vi "Main.vi"() -> ()   [LabVIEW 2023]
doc: "This template is for the Queued Message Handler design pattern.\n\nThe Event Handling Loop generates messages based on user interface actions.\n\nThe Message Handling Loop processes messages generated by the Event Handling Loop, or by other messages. The messages are string values, so new messages can be added easily to the Message Cases case structure in the Message Handling Loop. Each message cluster can also provide an optional value for Message Data, which is a variant that can be converted to whatever message-specific data is required."
uses:
  controls/JogParameters.ctl
  controls/MoveParameters.ctl
  controls/UI Data.ctl
  support/Message Queue/Enqueue Message (Single).vi
  chem-maldonado-motion-controller-api/GlobalVarsNetwork.vi
  <vilib>/Utility/error.llb/Error Cluster From Error Code.vi
  <vilib>/ErrorRing/Error Ring.xnode
  support/Message Queue/Message Queue.lvlib
  support/User Event - Stop/User Event - Stop.lvlib
panel:
  in  "Perform Home Routine":T1
  in  "Change Encoder Direction":T2
  out "Encoder Directions":T3
  out "X position (µm)":dbl
  out "X position (mm)":dbl
  out "Y position (µm)":dbl
  out "Y position (mm)":dbl
  out "Z position (µm)":dbl
  out "Z position (mm)":dbl
  in  "Jog Z":T4 {"Speed" min=0.0 max=1500.0}
  in  "Jog Y":T4 {"Speed" min=0.0 max=1500.0}
  in  "Move Z":T5 {"Speed" min=0.0 max=1500.0}
  in  "Move Y":T5 {"Speed" min=0.0 max=1500.0}
  in  "Move X":T5 {"Speed" min=0.0 max=1500.0}
  in  "Jog X":T4 {"Speed" min=0.0 max=1500.0}
  in  "Stop Motion":bool
  out "Action":string
  in  "Exit VI":bool
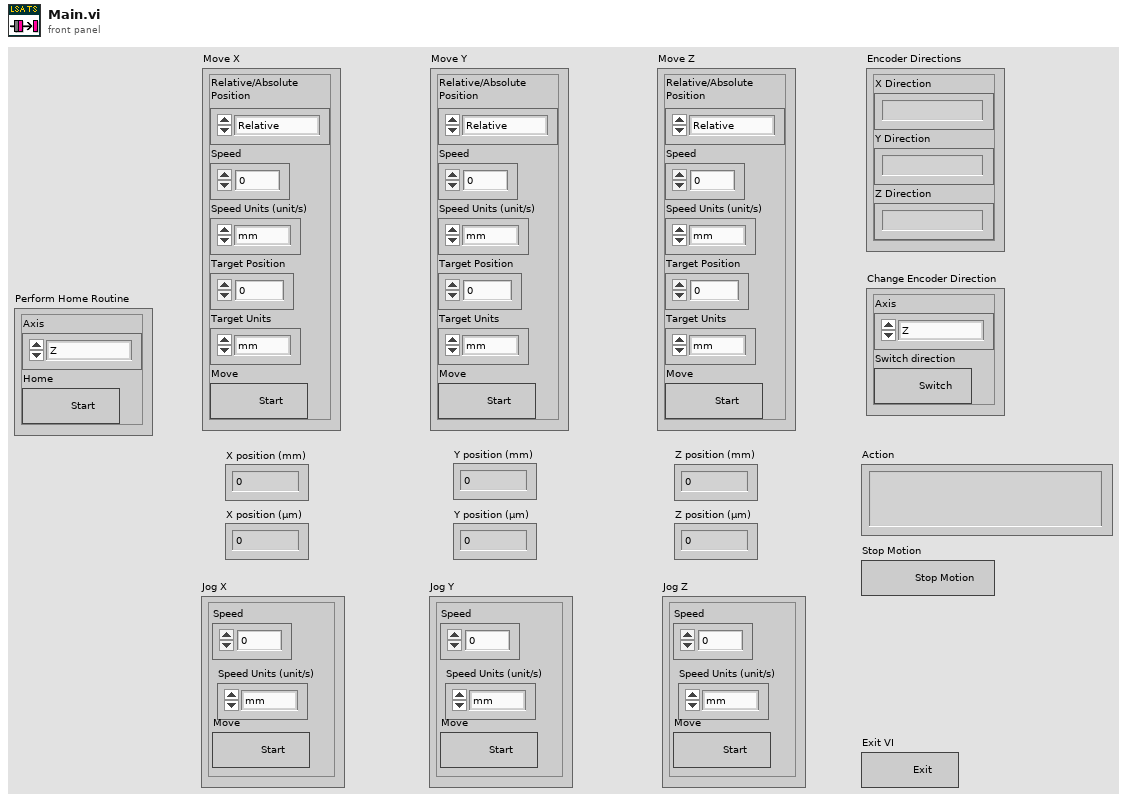
[diagram p1: front panel]
types:
  T1 = cluster{"Axis":enum16{"Z", "Y", "X"}, "Home":bool}
  T2 = cluster{"Axis":enum16{"Z", "Y", "X"}, "Switch direction":bool}
  T3 = cluster{"X Direction":string, "Y Direction":string, "Z Direction":string}
  T4 = typedef "JogParameters.ctl" = cluster{"Speed":dbl, "Speed Units (unit/s)":enum16{"mm", "µm"}, "Move":bool}
  T5 = typedef "MoveParameters.ctl" = cluster{"Relative/Absolute\nPosition":enum16{"Relative", "Absolute"}, "Speed":dbl, "Speed Units (unit/s)":enum16{"mm", "µm"}, "Target Position":dbl, "Target Units":enum16{"mm", "µm"}, "Move":bool}
  T6 = typedef "UI Data.ctl" = cluster{"Boolean <Replace Me>":bool, "String <Replace Me>":string, "Numeric <Replace Me>":dbl, "Do Something Ref":refnum<vi>, "Do Something Else Ref":refnum<vi>, "Data Display Ref":refnum<vi>, "Exit Button Ref":refnum<vi>, "StopMotion Button Ref":refnum<vi>}
  T7 = typedef "Message Queue.lvlib/All Message Queues.ctl" = cluster{"UI":refnum<queue>}
  T8 = cluster{"XY_IP_ADDRESS":string, "Z_IP_ADDRESS":string, "Port":u16, "connection refnum x,y":refnum<k5>, "connection refnum z":refnum<k5>}
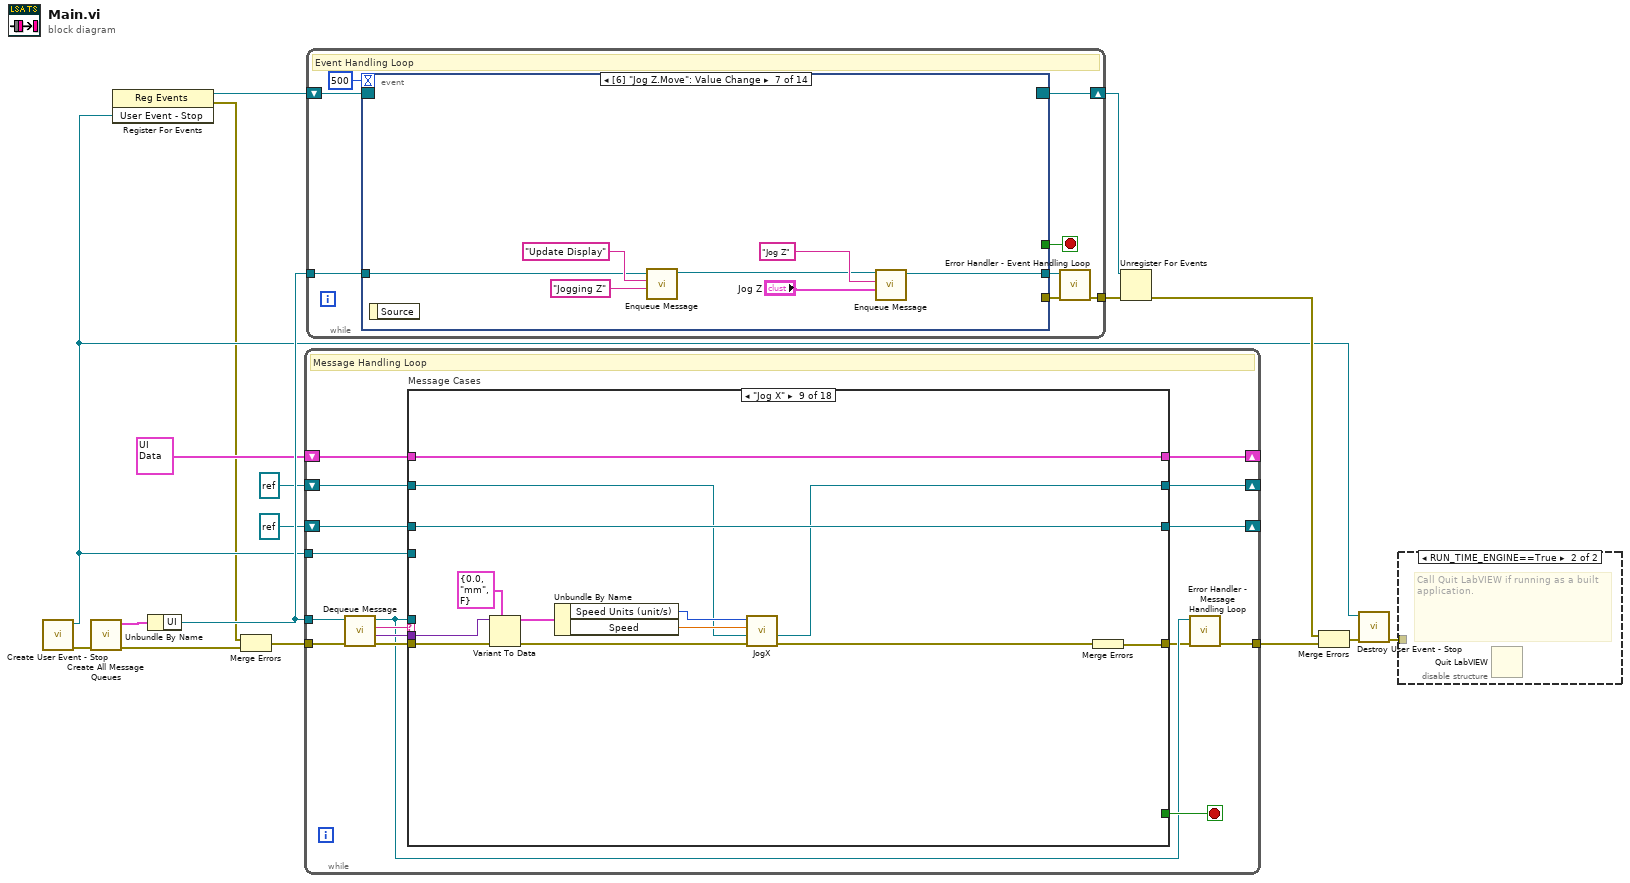
[diagram p0: block diagram]
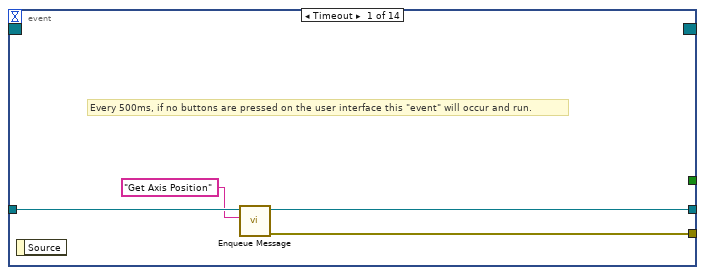
[diagram p3: hidden frame]
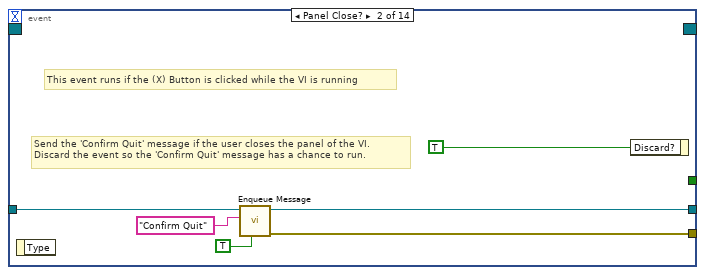
[diagram p4: hidden frame]
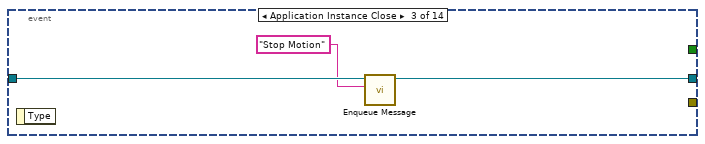
[diagram p5: hidden frame]
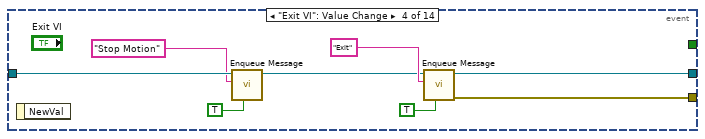
[diagram p6: hidden frame]
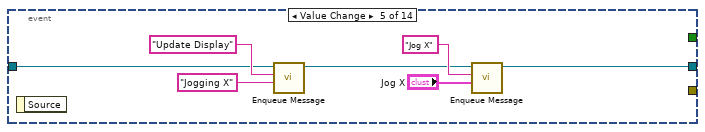
[diagram p7: hidden frame]
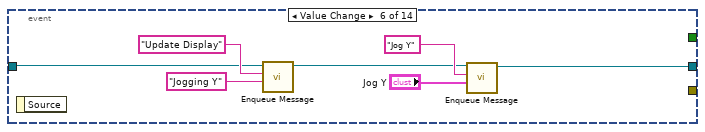
[diagram p8: hidden frame]
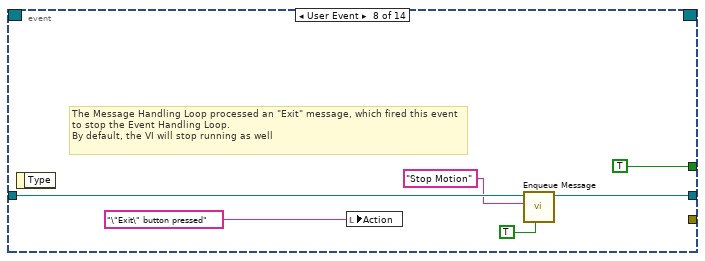
[diagram p9: hidden frame]
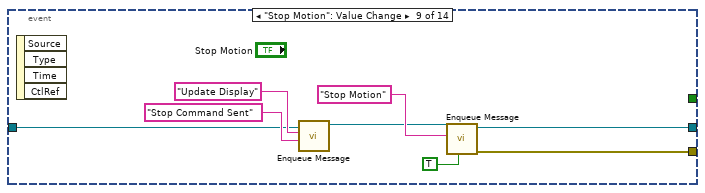
[diagram p10: hidden frame]
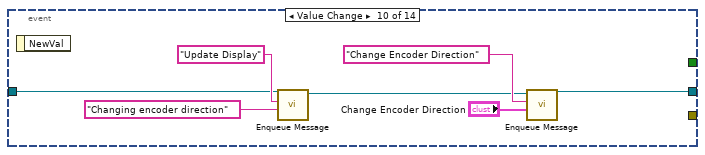
[diagram p11: hidden frame]
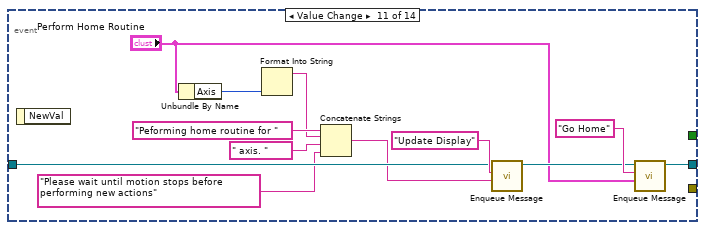
[diagram p12: hidden frame]
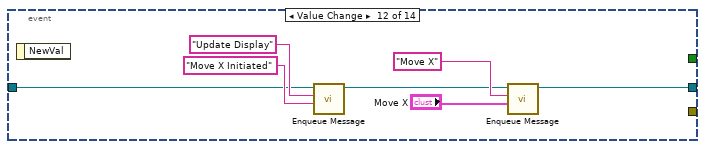
[diagram p13: hidden frame]
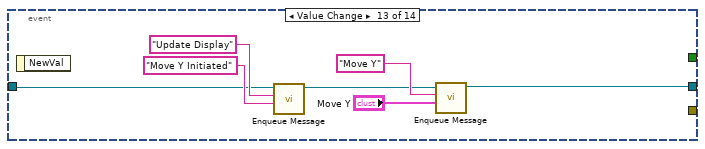
[diagram p14: hidden frame]
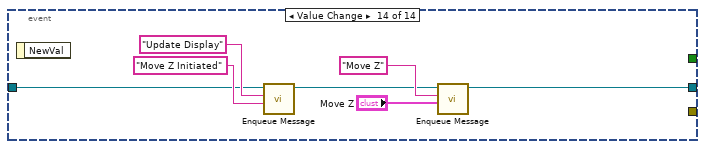
[diagram p15: hidden frame]
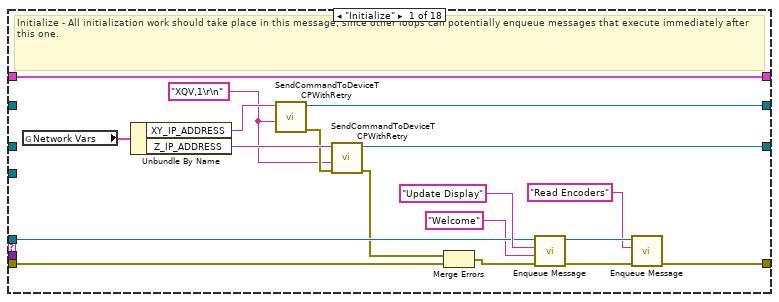
[diagram p16: hidden frame]
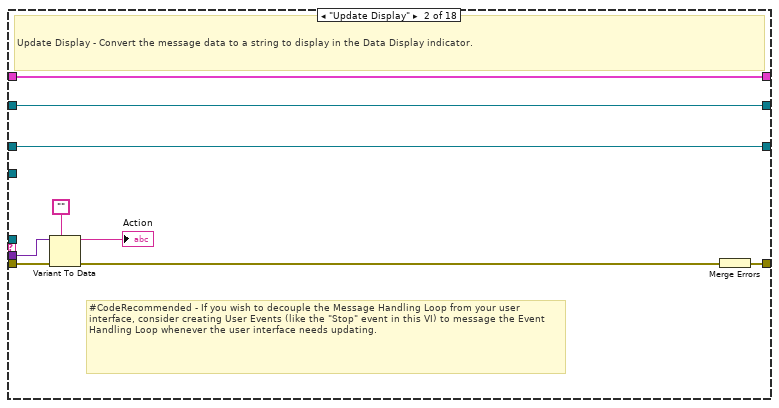
[diagram p17: hidden frame]
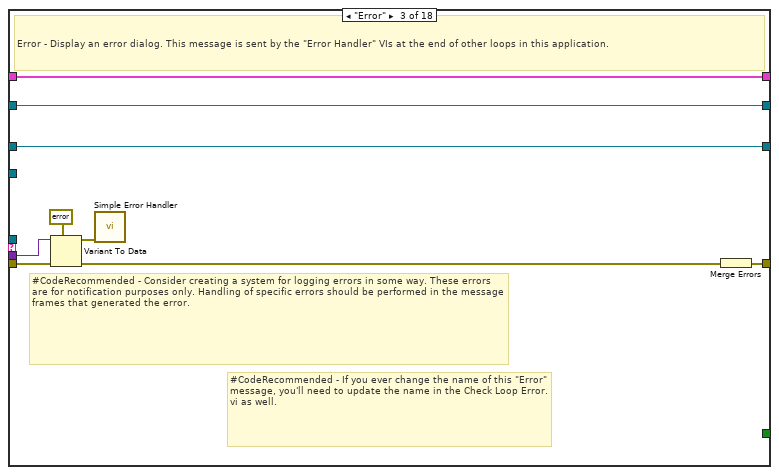
[diagram p18: hidden frame]
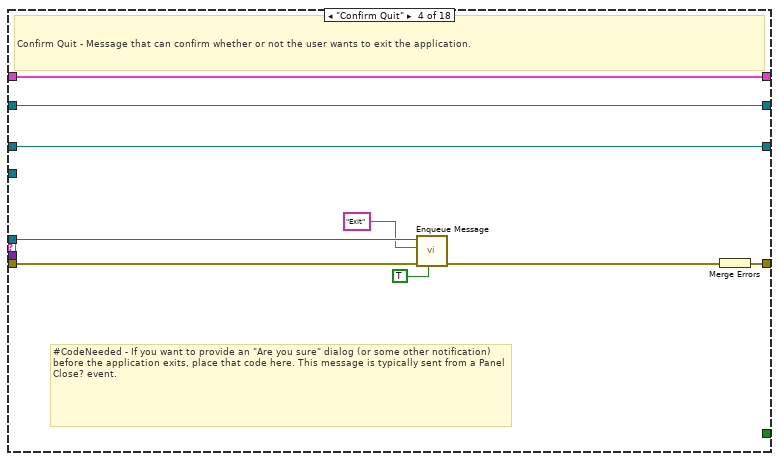
[diagram p19: hidden frame]
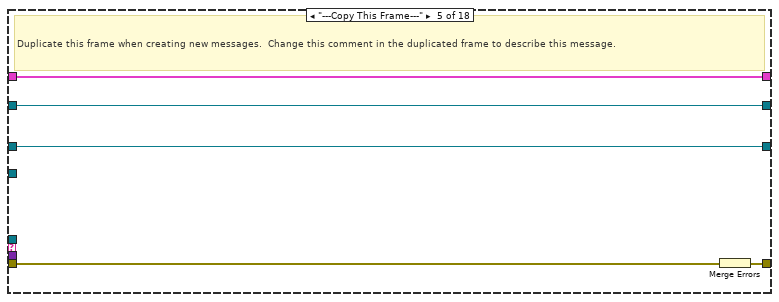
[diagram p20: hidden frame]
diagram:
  n1 = call "Create User Event - Stop.vi"() -> ("error out"=w13:errorcluster, "User Event - Stop"=w5:refnum<user-event>)  [unwired: 10 in]
  n2 = call "Create All Message Queues.vi"("error in (no error)"=w13) -> ("error out"=w17:errorcluster, "Message Queues out"=w16:T7)  [unwired: 9 in]
  n3 = register-events(w5) -> (reference out=w6:refnum<event-registration>, error out=w3:errorcluster)  [unwired: 2 in]
  n4 = Unbundle By Name(w16) -> ("UI"=w14:refnum<queue>)
  n5 = Merge Errors(w3, w17) -> (w4:errorcluster)
  n6 = while {
    tunnel: w14 -> [w25]
    shift-right: [w32] -> _
    shift-left: T6 {"Boolean <Replace Me>"=FALSE, "String <Replace Me>"="", "Numeric <Replace Me>"=0.0, "Do Something Ref"=refnum, "Do Something Else Ref"=refnum, "Data Display Ref"=refnum, "Exit Button Ref"=refnum, "StopMotion Button Ref"=refnum} ("Data Cluster") -> [w33]
    tunnel: w5 -> [w30]
    tunnel: w4 -> [w29]
    tunnel: [w23] -> w15
    shift-right: [w21] -> _
    shift-left: refnum<k5> refnum ("connection refnum out") -> [w20]
    shift-right: [w19] -> _
    shift-left: refnum<k5> refnum ("connection refnum out") -> [w18]
    stop <- w31 stop-if-true
    # "Message Handling Loop"
    n7 = call "Dequeue Message.vi"("error in (no error)"=w29, "Message Queue"=w25) -> ("error out"=w28:errorcluster, "Message Data"=w26:variant, "Message"=w27:string, "dup Message Queue"=w24:refnum<queue>)  [unwired: 6 in]
    n8 = case "Message Cases" shown="\"Jog X\"" w27 {
      selector: w27 -> [_ _ _ _ _ _ _ _ _ _ _ _ _ _ _ _ w302 _]
      tunnel: w24 -> [w50 _ _ w74 _ _ _ _ _ _ _ _ w199 w229 _ w299 _ _]
      tunnel: w28 -> [w42 w58 w69 w78 w83 w91 w105 w127 w142 w152 w165 w190 w205 w233 w265 w292 _ w318]
      tunnel: [w36 w59 w63 w76 w81 w88 w104 w129 w135 w148 w161 w189 w200 w235 w249 w295 w303 w317] -> w22
      tunnel: w33 -> [w48 w60 w68 w77 w82 w99 w114 w130 w143 w156 w169 w191 w217 w236 w266 w298 w304 w319]
      tunnel: [w48 w60 w68 w77 w82 w99 w114 w130 w143 w156 w169 w191 w217 w236 w266 w298 w304 w319] -> w32
      tunnel: [_ _ _ _ _ _ _ _ _ _ _ _ _ _ _ TRUE _ _] -> w31
      tunnel: w26 -> [_ w57 w67 _ _ w98 w112 w126 w139 w155 w166 _ _ w232 w263 w289 _ _]
      tunnel: w30 -> [_ _ _ _ _ _ _ _ _ _ _ _ _ _ _ w294 _ _]
      tunnel: [w40 w53 w62 w71 w80 w84 w100 w116 w131 w144 w157 w170 w207 w219 w253 w285 w300 w313] -> w21
      tunnel: w20 -> [_ w53 w62 w71 w80 w85 w101 w116 w132 w145 w157 w171 w209 w227 w256 w288 w300 w314]
      tunnel: [w39 w52 w61 w70 w79 w86 w102 w115 w133 w146 w158 w173 w206 w218 w251 w286 w301 w312] -> w19
      tunnel: w18 -> [_ w52 w61 w70 w79 w86 w102 w117 w133 w146 w159 w174 w210 w226 w252 w287 w301 w315]
      frame "Initialize" {
        w43 = "XQV,1\r\n" ("str command")
        # "Initialize - All initialization work should take place in this message, since other loops can potentially enqueue messages that execute immediately after this one."
        n9 = global read "GlobalVarsNetwork.vi" "Network Vars"() -> (w47:T8)
        n10 = Unbundle By Name(w47) -> ("XY_IP_ADDRESS"=w46:string, "Z_IP_ADDRESS"=w45:string)
        n11 = call "SendCommandToDeviceTCPWithRetry.vi"("str command"=w43, "IP address"=w46) -> ("error out"=w44:errorcluster, "connection refnum out"=w40:refnum<k5>)  [unwired: 6 in, 2 out]
        n12 = call "SendCommandToDeviceTCPWithRetry.vi"("error in"=w44, "str command"=w43, "IP address"=w45) -> ("error out"=w38:errorcluster, "connection refnum out"=w39:refnum<k5>)  [unwired: 5 in, 2 out]
        n13 = Merge Errors(w38, w42) -> (w41:errorcluster)
        n14 = call-poly "Enqueue Message.vi"("error in (no error)"=w41, "Message Data"="Welcome" ("Initial Message"), "Message"="Update Display", "Message Queue"=w50) -> ("error out"=w37:errorcluster, "dup Message Queue"=w35:refnum<queue>)  [unwired: 6 in]
        n15 = call-poly "Enqueue Message.vi"("error in (no error)"=w37, "Message"="Read Encoders", "Message Queue"=w35) -> ("error out"=w36:errorcluster)  [unwired: 7 in, 1 out]
      }
      frame "Update Display" {
        # "#CodeRecommended - If you wish to decouple the Message Handling Loop from your user interface, consider creating User Events (like the \"Stop\" event in this VI) to message the Event Handling Loop whenever the user interface needs updating."
        # "Update Display - Convert the message data to a string to display in the Data Display indicator."
        n16 = Variant To Data(error in=w58, type="", Variant=w57) -> (data=→"Action":string, error out=w55:errorcluster)
        n17 = Merge Errors(w55) -> (w59:errorcluster)
      }
      frame "Error" {
        # "#CodeRecommended - If you ever change the name of this \"Error\" message, you'll need to update the name in the Check Loop Error.vi as well."
        # "#CodeRecommended - Consider creating a system for logging errors in some way. These errors are for notification purposes only. Handling of specific errors should be performed in the message frames that generated the error."
        # "Error - Display an error dialog. This message is sent by the \"Error Handler\" VIs at the end of other loops in this application."
        n18 = Variant To Data(error in=w69, type=errorcluster {"status"=FALSE, "code"=0, "source"=""} ("error constant"), Variant=w67) -> (data=w65:errorcluster, error out=w64:errorcluster)
        n19 = call <vilib>:"Simple Error Handler.vi"("error in (no error)"=w65) -> ()  [unwired: 4 in, 5 out]
        n20 = Merge Errors(w64) -> (w63:errorcluster)
      }
      frame "Confirm Quit" {
        # "#CodeNeeded - If you want to provide an \"Are you sure\" dialog (or some other notification) before the application exits, place that code here. This message is typically sent from a Panel Close? event."
        # "Confirm Quit - Message that can confirm whether or not the user wants to exit the application."
        n21 = call-poly "Enqueue Message.vi"("Priority Message? (F)"=TRUE, "error in (no error)"=w78, "Message"="Exit", "Message Queue"=w74) -> ("error out"=w75:errorcluster)  [unwired: 6 in, 1 out]
        n22 = Merge Errors(w75) -> (w76:errorcluster)
      }
      frame "---Copy This Frame---" {
        # "Duplicate this frame when creating new messages.  Change this comment in the duplicated frame to describe this message."
        n23 = Merge Errors(w83) -> (w81:errorcluster)
      }
      frame "Move X" {
        n24 = Variant To Data(error in=w91, type=T5 {"Relative/Absolute\nPosition"=enum."Relative", "Speed"=0.0, "Speed Units (unit/s)"=enum."mm", "Target Position"=0.0, "Target Units"=enum."mm", "Move"=FALSE} ("Move Parameters X"), Variant=w98) -> (data=w97:T5, error out=w90:errorcluster)
        n25 = Unbundle By Name(w97) -> ("Relative/Absolute\nPosition"=w96:enum16{"Relative", "Absolute"}, "Speed"=w95:dbl, "Speed Units (unit/s)"=w94:enum16{"mm", "µm"}, "Target Position"=w93:dbl, "Target Units"=w92:enum16{"mm", "µm"})
        n26 = call "MoveX.vi"("Speed (units/s)"=w95, "Relative/Absolute\nPosition"=w96, "connection refnum in"=w85, "Speed Units"=w94, "Target Position"=w93, "Target Units"=w92, "error in"=w90) -> ("connection refnum out xy"=w84:refnum<k5>, "error out"=w87:errorcluster)  [unwired: 6 in, 1 out]
        n27 = Merge Errors(w87) -> (w88:errorcluster)
      }
      frame "Move Y" {
        # "Duplicate this frame when creating new messages.  Change this comment in the duplicated frame to describe this message."
        n28 = Variant To Data(type=T5 {"Relative/Absolute\nPosition"=enum."Relative", "Speed"=0.0, "Speed Units (unit/s)"=enum."mm", "Target Position"=0.0, "Target Units"=enum."mm", "Move"=FALSE} ("Move Parameters Y"), Variant=w112) -> (data=w111:T5)  [unwired: 1 in, 1 out]
        n29 = Unbundle By Name(w111) -> ("Relative/Absolute\nPosition"=w110:enum16{"Relative", "Absolute"}, "Speed"=w109:dbl, "Speed Units (unit/s)"=w108:enum16{"mm", "µm"}, "Target Position"=w107:dbl, "Target Units"=w106:enum16{"mm", "µm"})
        n30 = call "MoveY.vi"("Speed (unit/s)"=w109, "Relative/Absolute\nPosition"=w110, "connection refnum in"=w101, "Speed Units"=w108, "Target Position"=w107, "Target Units"=w106, "error in"=w105) -> ("connection refnum out xy"=w100:refnum<k5>, "error out"=w103:errorcluster)  [unwired: 6 in, 1 out]
        n31 = Merge Errors(w103) -> (w104:errorcluster)
      }
      frame "Move Z" {
        # "Duplicate this frame when creating new messages.  Change this comment in the duplicated frame to describe this message."
        n32 = Variant To Data(error in=w127, type=T5 {"Relative/Absolute\nPosition"=enum."Relative", "Speed"=0.0, "Speed Units (unit/s)"=enum."mm", "Target Position"=0.0, "Target Units"=enum."mm", "Move"=FALSE} ("Move Parameters Z"), Variant=w126) -> (data=w125:T5, error out=w119:errorcluster)
        n33 = Unbundle By Name(w125) -> ("Relative/Absolute\nPosition"=w124:enum16{"Relative", "Absolute"}, "Speed"=w123:dbl, "Speed Units (unit/s)"=w122:enum16{"mm", "µm"}, "Target Position"=w121:dbl, "Target Units"=w120:enum16{"mm", "µm"})
        n34 = call "MoveZ.vi"("Speed (unit/s)"=w123, "Relative/Absolute\nPosition"=w124, "connection refnum in"=w117, "Speed Units"=w122, "Target Position"=w121, "Target Units"=w120, "error in"=w119) -> ("connection refnum out z"=w115:refnum<k5>, "error out"=w118:errorcluster)  [unwired: 6 in, 1 out]
        n35 = Merge Errors(w118) -> (w129:errorcluster)
      }
      frame "Jog X" {
        n36 = Variant To Data(error in=w142, type=T4 {"Speed"=0.0, "Speed Units (unit/s)"=enum."mm", "Move"=FALSE} ("Jog X"), Variant=w139) -> (data=w138:T4, error out=w141:errorcluster)
        n37 = Unbundle By Name(w138) -> ("Speed Units (unit/s)"=w136:enum16{"mm", "µm"}, "Speed"=w137:dbl)
        n38 = call "JogX.vi"("error in"=w141, "connection refnum in"=w132, "Speed (units/s)"=w137, "Units"=w136) -> ("error out"=w134:errorcluster, "connection refnum out"=w131:refnum<k5>)  [unwired: 6 in]
        n39 = Merge Errors(w134) -> (w135:errorcluster)
      }
      frame "Jog Y" {
        n40 = Variant To Data(error in=w152, type=T4 {"Speed"=0.0, "Speed Units (unit/s)"=enum."mm", "Move"=FALSE} ("Jog X"), Variant=w155) -> (data=w153:T4, error out=w149:errorcluster)
        n41 = Unbundle By Name(w153) -> ("Speed Units (unit/s)"=w150:enum16{"mm", "µm"}, "Speed"=w151:dbl)
        n42 = call "JogY.vi"("error in"=w149, "connection refnum in"=w145, "Speed (units/s)"=w151, "Units"=w150) -> ("error out"=w147:errorcluster, "connection refnum out xy"=w144:refnum<k5>)  [unwired: 6 in]
        n43 = Merge Errors(w147) -> (w148:errorcluster)
      }
      frame "Jog Z" {
        n44 = Variant To Data(error in=w165, type=T4 {"Speed"=0.0, "Speed Units (unit/s)"=enum."mm", "Move"=FALSE} ("Jog X"), Variant=w166) -> (data=w168:T4, error out=w164:errorcluster)
        n45 = Unbundle By Name(w168) -> ("Speed Units (unit/s)"=w162:enum16{"mm", "µm"}, "Speed"=w163:dbl)
        n46 = call "JogZ.vi"("error in"=w164, "connection refnum in"=w159, "Speed (units/s)"=w163, "Units"=w162) -> ("error out"=w160:errorcluster, "connection refnum out z"=w158:refnum<k5>)  [unwired: 6 in]
        n47 = Merge Errors(w160) -> (w161:errorcluster)
      }
      frame "Get Axis Position" {
        n48 = call "GetAxisPosition.vi"("Axis"=enum16{"Z", "Y", "X"}."Z", "connection refnum in"=w174, "error in"=w190) -> ("connection refnum out"=w173:refnum<k5>, "numeric result"=w186:i32, "error out"=w188:errorcluster)  [unwired: 1 out]
        n49 = call "CountsToUnit.vi"("Counts"=w186) -> ("mm"=→"Z position (mm)":dbl, "µm"=→"Z position (µm)":dbl)  [unwired: 1 in, 1 out]
        n50 = call "GetAxisPosition.vi"("Axis"=enum16{"Z", "Y", "X"}."Y", "connection refnum in"=w171, "error in"=w188) -> ("connection refnum out"=w172:refnum<k5>, "numeric result"=w185:i32, "error out"=w187:errorcluster)  [unwired: 1 out]
        n51 = call "CountsToUnit.vi"("Counts"=w185) -> ("mm"=→"Y position (mm)":dbl, "µm"=→"Y position (µm)":dbl)  [unwired: 1 in, 1 out]
        n52 = call "GetAxisPosition.vi"("Axis"=enum16{"Z", "Y", "X"}."X", "connection refnum in"=w172, "error in"=w187) -> ("connection refnum out"=w170:refnum<k5>, "numeric result"=w184:i32, "error out"=w189:errorcluster)  [unwired: 1 out]
        n53 = call "CountsToUnit.vi"("Counts"=w184) -> ("mm"=→"X position (mm)":dbl, "µm"=→"X position (µm)":dbl)  [unwired: 1 in, 1 out]
      }
      frame "Read Encoders" {
        n54 = global read "GlobalVarsNetwork.vi" "Network Vars"() -> (w196:T8)
        n55 = Unbundle By Name(w196) -> ("XY_IP_ADDRESS"=w195:string, "Z_IP_ADDRESS"=w194:string)
        n56 = call "ReadEncoderDirection.vi"("error in"=w205, "IP address"=w195, "Axis"=enum16{"Z", "Y", "X"}."X", "connection refnum in"=w209) -> ("error out"=w216:errorcluster, "Encoder Direction"=w204:string, "connection refnum out"=w208:refnum<k5>)  [unwired: 4 in, 1 out]
        n57 = call "ReadEncoderDirection.vi"("error in"=w216, "IP address"=w195, "Axis"=enum16{"Z", "Y", "X"}."Y", "connection refnum in"=w208) -> ("error out"=w215:errorcluster, "Encoder Direction"=w203:string, "connection refnum out"=w207:refnum<k5>)  [unwired: 4 in, 1 out]
        n58 = call "ConvertZAxisToX.vi"("Axis in"=enum16{"Z", "Y", "X"}."Z" ("Axis")) -> ("Axis out"=w192:enum16{"Z", "Y", "X"})  [unwired: 6 in]
        n59 = call "ReadEncoderDirection.vi"("error in"=w215, "IP address"=w194, "Axis"=w192, "connection refnum in"=w210) -> ("error out"=w201:errorcluster, "Encoder Direction"=w202:string, "connection refnum out"=w206:refnum<k5>)  [unwired: 4 in, 1 out]
        n60 = Bundle By Name(cluster=T3 {"X Direction"="", "Y Direction"="", "Z Direction"=""} ("Encoder Directions"), "X Direction"=w204, "Y Direction"=w203, "Z Direction"=w202) -> (→"Encoder Directions":T3)
        n61 = call-poly "Enqueue Message.vi"("error in (no error)"=w201, "Message Data"="Encoder values updated" ("Message"), "Message"="Update Display", "Message Queue"=w199) -> ("error out"=w200:errorcluster)  [unwired: 6 in, 1 out]
      }
      frame "Change Encoder Direction" {
        n62 = Variant To Data(error in=w233, type=T2 {"Axis"=enum."Z", "Switch direction"=FALSE} ("Change Encoder Direction"), Variant=w232) -> (data=w230:T2, error out=w224:errorcluster)
        n63 = Unbundle By Name(w230) -> ("Axis"=w228:enum16{"Z", "Y", "X"})  [unwired: 1 out]
        n64 = case shown="\"Y\", \"X\"" w228 {
          selector: w228 -> [w245 w248]
          tunnel: w227 -> [w243 w247]
          tunnel: [w244 w247] -> w225
          tunnel: w226 -> [w244 w246]
          tunnel: [w245 w248] -> w222
          tunnel: [w243 w246] -> w220
          frame "Z", Default {
          }
          frame "Y", "X" {
          }
        }
        n65 = call "ReverseEncoderDirection.vi"("error in"=w224, "Axis"=w222, "connection refnum in"=w225) -> ("error out"=w223:errorcluster, "connection refnum out"=w221:refnum<k5>)  [unwired: 6 in, 1 out]
        n66 = case shown="\"Z\", Default" w222 {
          selector: w222 -> [w239 w242]
          tunnel: [w239 w242] -> _
          tunnel: w221 -> [w237 w241]
          tunnel: w220 -> [w238 w240]
          tunnel: [w238 w241] -> w219
          tunnel: [w237 w240] -> w218
          frame "Z", Default {
          }
          frame "Y", "X" {
          }
        }
        n67 = call-poly "Enqueue Message.vi"("error in (no error)"=w223, "Message"="Read Encoders", "Message Queue"=w229) -> ("error out"=w235:errorcluster)  [unwired: 7 in, 1 out]
      }
      frame "Go Home" {
        n68 = Variant To Data(error in=w265, type=T1 {"Axis"=enum."Z", "Home"=FALSE} ("Perform Home Routine"), Variant=w263) -> (data=w262:T1, error out=w260:errorcluster)
        n69 = Unbundle By Name(w262) -> ("Axis"=w261:enum16{"Z", "Y", "X"})
        n70 = case shown="\"Z\", Default" w261 {
          selector: w261 -> [w278 w282]
          tunnel: [w278 w282] -> w257
          tunnel: w260 -> [w275 w281]
          tunnel: [w275 w281] -> w259
          tunnel: w256 -> [w277 w280]
          tunnel: [w276 w280] -> w255
          tunnel: w252 -> [w276 w279]
          tunnel: [w277 w279] -> w250
          frame "Z", Default {
          }
          frame "Y", "X" {
          }
        }
        n71 = call "GoHome.vi"("error in"=w259, "Axis"=w257, "connection refnum in"=w255) -> ("error out"=w258:errorcluster, "connection refnum out"=w254:refnum<k5>)  [unwired: 1 in]
        n72 = case shown="\"Z\", Default" w257 {
          selector: w257 -> [w270 w274]
          tunnel: [w270 w274] -> _
          tunnel: w258 -> [w267 w273]
          tunnel: [w267 w273] -> w249
          tunnel: w254 -> [w269 w272]
          tunnel: [w268 w272] -> w253
          tunnel: [w269 w271] -> w251
          tunnel: w250 -> [w268 w271]
          frame "Z", Default {
          }
          frame "Y", "X" {
          }
        }
      }
      frame "Exit" {
        # "Stop the VI"
        # "Release the message queue reference"
        # "#CodeNeeded - Add any required cleanup code here. Note that if 'Exit' was called as a result of an error, an error dialog will be displayed. Add any custom error handling for an 'Exit' condition here as well."
        # "Exit - Exit the application."
        n73 = Variant To Data(type=errorcluster {"status"=FALSE, "code"=0, "source"=""} ("error constant"), Variant=w289) -> (data=w290:errorcluster)  [unwired: 1 in, 1 out]
        n74 = call <vilib>:"Simple Error Handler.vi"("error in (no error)"=w290) -> ()  [unwired: 4 in, 5 out]
        n75 = call "Fire User Event - Stop.vi"("User Event - Stop"=w294) -> ("error out"=w293:errorcluster)  [unwired: 10 in]
        n76 = Release Queue(queue=w299, error in (no error)=w292) -> (error out=w296:errorcluster)  [unwired: 1 in, 2 out]
        n77 = TCP Close Connection(connection ID=w288) -> (connection ID out=w285:refnum<k5>, error out=w283:errorcluster)  [unwired: 2 in]
        n78 = TCP Close Connection(connection ID=w287) -> (connection ID out=w286:refnum<k5>, error out=w284:errorcluster)  [unwired: 2 in]
        n79 = Merge Errors(w283, w284, w293, w296) -> (w295:errorcluster)
      }
      frame Default {
        # "'Default' case only runs if there is a message that isn't defined in any of the other cases.  Output a programming error."
        n80 = xnode "Error Ring"("parameter 0"=w302) -> ("error out"=w303:errorcluster)
      }
      frame "Stop Motion" {
        n81 = call "StopMove.vi"("error in"=w318, "Stop?"=TRUE, "connection refnum in,  z"=w315, "connection refnum in, xy"=w314) -> ("error out"=w317:errorcluster, "connection refnum out z"=w312:refnum<k5>, "connection refnum out xy"=w313:refnum<k5>)  [unwired: 1 out]
      }
    }
    n82 = call "Error Handler - Message Handling Loop.vi"("error in (no error)"=w22, "Message Queue"=w24) -> ("dup error in"=w23:errorcluster)  [unwired: 8 in, 1 out]
  }
  n83 = while {
    tunnel: w14 -> [w327]
    shift-right: [w325] -> w10
    shift-left: w6 -> [w326]
    tunnel: [w321] -> w7
    stop <- w323 stop-if-true
    # "Event Handling Loop"
    n84 = event shown="[6] \"Jog Z.Move\": Value Change" {
      selector: w326 -> [_ _ _ _ _ _ _ _ _ _ _ _ _ _]
      dyn-events: [_ _ _ _ _ _ _ _ _ _ _ _ _ _] -> w325
      timeout: 500 -> [_ _ _ _ _ _ _ _ _ _ _ _ _ _]
      tunnel: [_ _ _ _ _ _ _ TRUE ("Discard?") _ _ _ _ _ _] -> w323
      tunnel: w327 -> [w331 w336 w340 w343 w350 w357 w364 w373 w378 w385 w399 w404 w411 w418]
      tunnel: [w329 w335 _ w348 _ _ _ _ w382 _ _ _ _ _] -> w324
      tunnel: [w330 w334 w338 w347 w355 w360 w368 w372 w383 w390 w402 w409 w416 w423] -> w322
      event Timeout {
        # "Every 500ms, if no buttons are pressed on the user interface this \"event\" will occur and run."
        n85 = event-data() -> ()  [unwired: 1 in, 1 out]
        n86 = call-poly "Enqueue Message.vi"("Message"="Get Axis Position", "Message Queue"=w331) -> ("error out"=w329:errorcluster, "dup Message Queue"=w330:refnum<queue>)  [unwired: 8 in]
      }
      event Panel Close? {
        # "This event runs if the (X) Button is clicked while the VI is running"
        # "Send the 'Confirm Quit' message if the user closes the panel of the VI. Discard the event so the 'Confirm Quit' message has a chance to run."
        n87 = event-data() -> ()  [unwired: 1 in, 1 out]
        n88 = call-poly "Enqueue Message.vi"("Priority Message? (F)"=TRUE, "Message"="Confirm Quit", "Message Queue"=w336) -> ("error out"=w335:errorcluster, "dup Message Queue"=w334:refnum<queue>)  [unwired: 7 in]
        n89 = event-data("Discard?"=TRUE) -> ()  [unwired: 1 in, 1 out]
      }
      event Application Instance Close {
        n90 = event-data() -> ()  [unwired: 1 in, 1 out]
        n91 = call-poly "Enqueue Message.vi"("Message"="Stop Motion", "Message Queue"=w340) -> ("dup Message Queue"=w338:refnum<queue>)  [unwired: 8 in, 1 out]
      }
      event "Exit VI": Value Change {
        n92 = event-data() -> ()  [unwired: 1 in, 1 out]
        n93 = call-poly "Enqueue Message.vi"("Priority Message? (F)"=TRUE, "Message"="Stop Motion", "Message Queue"=w343) -> ("dup Message Queue"=w342:refnum<queue>)  [unwired: 7 in, 1 out]
        n94 = call-poly "Enqueue Message.vi"("Priority Message? (F)"=TRUE, "Message"="Exit", "Message Queue"=w342) -> ("error out"=w348:errorcluster, "dup Message Queue"=w347:refnum<queue>)  [unwired: 7 in]
      }
      event Value Change {
        n95 = event-data() -> ()  [unwired: 1 in, 1 out]
        n96 = call-poly "Enqueue Message.vi"("Message Data"="Jogging X" ("Message"), "Message"="Update Display", "Message Queue"=w350) -> ("dup Message Queue"=w349:refnum<queue>)  [unwired: 7 in, 1 out]
        n97 = call-poly "Enqueue Message.vi"("Message Data"="Jog X", "Message"="Jog X", "Message Queue"=w349) -> ("dup Message Queue"=w355:refnum<queue>)  [unwired: 7 in, 1 out]
      }
      event Value Change {
        n98 = event-data() -> ()  [unwired: 1 in, 1 out]
        n99 = call-poly "Enqueue Message.vi"("Message Data"="Jogging Y" ("Message"), "Message"="Update Display", "Message Queue"=w357) -> ("dup Message Queue"=w356:refnum<queue>)  [unwired: 7 in, 1 out]
        n100 = call-poly "Enqueue Message.vi"("Message Data"="Jog Y", "Message"="Jog Y", "Message Queue"=w356) -> ("dup Message Queue"=w360:refnum<queue>)  [unwired: 7 in, 1 out]
      }
      event Value Change {
        n101 = event-data() -> ()  [unwired: 1 in, 1 out]
        n102 = call-poly "Enqueue Message.vi"("Message Data"="Jogging Z" ("Message"), "Message"="Update Display", "Message Queue"=w364) -> ("dup Message Queue"=w363:refnum<queue>)  [unwired: 7 in, 1 out]
        n103 = call-poly "Enqueue Message.vi"("Message Data"="Jog Z", "Message"="Jog Z", "Message Queue"=w363) -> ("dup Message Queue"=w368:refnum<queue>)  [unwired: 7 in, 1 out]
      }
      event User Event {
        # "The Message Handling Loop processed an \"Exit\" message, which fired this event to stop the Event Handling Loop.\nBy default, the VI will stop running as well"
        n104 = event-data() -> ()  [unwired: 1 in, 1 out]
        n105 = local write "Action"("\"Exit\" button pressed" ("VI Stopped")) -> ()
        n106 = call-poly "Enqueue Message.vi"("Priority Message? (F)"=TRUE, "Message"="Stop Motion", "Message Queue"=w373) -> ("dup Message Queue"=w372:refnum<queue>)  [unwired: 7 in, 1 out]
      }
      event "Stop Motion": Value Change {
        n107 = event-data() -> ()  [unwired: 1 in, 4 out]
        n108 = call-poly "Enqueue Message.vi"("Message Data"="Stop Command Sent" ("Message"), "Message"="Update Display", "Message Queue"=w378) -> ("dup Message Queue"=w377:refnum<queue>)  [unwired: 7 in, 1 out]
        n109 = call-poly "Enqueue Message.vi"("Priority Message? (F)"=TRUE, "Message"="Stop Motion", "Message Queue"=w377) -> ("error out"=w382:errorcluster, "dup Message Queue"=w383:refnum<queue>)  [unwired: 7 in]
      }
      event "Change Encoder Direction.Switch direction": Value Change {
        n110 = event-data() -> ()  [unwired: 1 in, 1 out]
        n111 = call-poly "Enqueue Message.vi"("Message Data"="Changing encoder direction" ("Message"), "Message"="Update Display", "Message Queue"=w385) -> ("dup Message Queue"=w384:refnum<queue>)  [unwired: 7 in, 1 out]
        n112 = call-poly "Enqueue Message.vi"("Message Data"="Change Encoder Direction", "Message"="Change Encoder Direction", "Message Queue"=w384) -> ("dup Message Queue"=w390:refnum<queue>)  [unwired: 7 in, 1 out]
      }
      event "Perform Home Routine.Home": Value Change {
        n113 = event-data() -> ()  [unwired: 1 in, 1 out]
        n114 = Unbundle By Name("Perform Home Routine") -> ("Axis"=w395:enum16{"Z", "Y", "X"})
        n115 = Format Into String(w395) -> (resulting string=w394:string)  [unwired: 3 in, 1 out]
        n116 = Concatenate Strings("Peforming home routine for " ("Message"), w394, " axis. " ("Message"), "Please wait until motion stops before performing new actions" ("Message")) -> (w392:string)
        n117 = call-poly "Enqueue Message.vi"("Message Data"=w392, "Message"="Update Display", "Message Queue"=w399) -> ("dup Message Queue"=w398:refnum<queue>)  [unwired: 7 in, 1 out]
        n118 = call-poly "Enqueue Message.vi"("Message Data"="Perform Home Routine", "Message"="Go Home", "Message Queue"=w398) -> ("dup Message Queue"=w402:refnum<queue>)  [unwired: 7 in, 1 out]
      }
      event Value Change {
        n119 = event-data() -> ()  [unwired: 1 in, 1 out]
        n120 = call-poly "Enqueue Message.vi"("Message Data"="Move X Initiated" ("Message"), "Message"="Update Display", "Message Queue"=w404) -> ("dup Message Queue"=w403:refnum<queue>)  [unwired: 7 in, 1 out]
        n121 = call-poly "Enqueue Message.vi"("Message Data"="Move X", "Message"="Move X", "Message Queue"=w403) -> ("dup Message Queue"=w409:refnum<queue>)  [unwired: 7 in, 1 out]
      }
      event Value Change {
        n122 = event-data() -> ()  [unwired: 1 in, 1 out]
        n123 = call-poly "Enqueue Message.vi"("Message Data"="Move Y Initiated" ("Message"), "Message"="Update Display", "Message Queue"=w411) -> ("dup Message Queue"=w410:refnum<queue>)  [unwired: 7 in, 1 out]
        n124 = call-poly "Enqueue Message.vi"("Message Data"="Move Y", "Message"="Move Y", "Message Queue"=w410) -> ("dup Message Queue"=w416:refnum<queue>)  [unwired: 7 in, 1 out]
      }
      event Value Change {
        n125 = event-data() -> ()  [unwired: 1 in, 1 out]
        n126 = call-poly "Enqueue Message.vi"("Message Data"="Move Z Initiated" ("Message"), "Message"="Update Display", "Message Queue"=w418) -> ("dup Message Queue"=w417:refnum<queue>)  [unwired: 7 in, 1 out]
        n127 = call-poly "Enqueue Message.vi"("Message Data"="Move Z", "Message"="Move Z", "Message Queue"=w417) -> ("dup Message Queue"=w423:refnum<queue>)  [unwired: 7 in, 1 out]
      }
    }
    n128 = call "Error Handler - Event Handling Loop.vi"("error in (no error)"=w324, "Message Queue"=w322) -> ("dup error in"=w321:errorcluster)  [unwired: 8 in, 1 out]
  }
  n129 = Unregister For Events(event registration refnum=w10, error in=w7) -> (error out=w11:errorcluster)
  n130 = Merge Errors(w11, w15) -> (w12:errorcluster)
  n131 = call "Destroy User Event - Stop.vi"("error in (no error)"=w12, "User Event - Stop"=w5) -> ("error out"=w8:errorcluster)  [unwired: 9 in]
  n132 = disable-structure shown="RUN_TIME_ENGINE==True" {
    disable-tunnel: w8 -> [_ _]
    frame condition #0 (active) {
    }
    frame condition #1 {
      # "Call Quit LabVIEW if running as a built application."
      n133 = Quit LabVIEW() -> ()  [unwired: 1 in]
    }
  }
